vi "Get Amp Desc.vi"(9 "length":i32, 10 "name":string, 11 "index":i32) -> (2 "name out":string, 3 "function return":u32)   [LabVIEW 2018, in "Copy of Andor SDK.lvlib"]
doc: "EXPNETTYPE unsigned int WINAPI GetAmpDesc(int index, char * name, int length);"
uses:
  Copy of Andor SDK.lvlib
  <userlib>/Andor SDK/ATMCD32D.dll
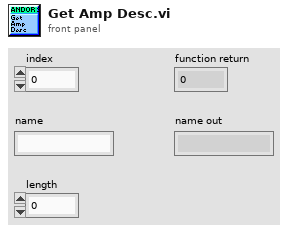
[diagram p1: front panel]
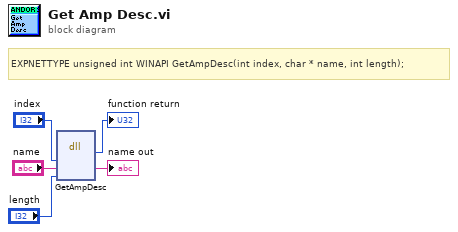
[diagram p0: block diagram]
diagram:
  # "EXPNETTYPE unsigned int WINAPI GetAmpDesc(int index, char * name, int length);"
  n1 = dll-call lib="C:/Program Files (x86)/National Instruments/LabVIEW 2018/user.lib/Andor SDK/ATMCD32D.*" fn="GetAmpDesc"("index"="index", "name"="name", "length"="length") -> (→"function return":u32, "name"=→"name out":string)  [unwired: 5 in, 2 out]
